vi "Run VI.vi"(1 "VI name":string, 2 "stripped path":path) -> ()   [LabVIEW 2017]
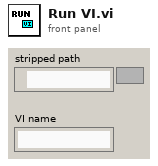
[diagram p1: front panel]
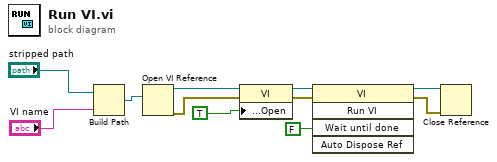
[diagram p0: block diagram]
diagram:
  n1 = Build Path(base path="stripped path", name or relative path="VI name") -> (appended path=w9:path)
  n2 = Open VI Reference(vi path=w9) -> (vi reference=w7:refnum<vi>, error out=w6:errorcluster)  [unwired: 5 in]
  n3 = property class="VI"(reference=w7, error in=w6, "Front Panel Window:Open"=TRUE) -> (reference out=w4:refnum<vi>, error out=w3:errorcluster)
  n4 = invoke class="VI" method="Run VI"(reference=w4, error in=w3, "Wait until done"=FALSE) -> (reference out=w1:refnum<vi>, error out=w2:errorcluster)  [unwired: 2 in, 3 out]
  n5 = Close Reference(reference=w1, error in (no error)=w2) -> ()  [unwired: 1 out]
